vi "Lidar Camera System.vi"() -> ()   [LabVIEW 2017]
doc: "This example project provides a library of VIs that work together to wrap various ethernet packet sniffing functions available from WinPcap, a Windows packet capture program.\n\nNote: You must install WinPcap before running this example. You can download WinPcap from www.winpcap.org.\n\nThis VI reads ethernet packets. It outputs the raw data for the packet as a hexadecimal string. It also parses out the ethernet and IP header information, as well as timestamp information for each packet.\n\nThis VI also enumerates all the ethernet adapters on your system and allows you interactively to select between the various adapters.\n\nPlease note that this project is for demonstration purposes only. It was designed to demonstrate one method in which LabVIEW can be used to interface with external software utilities (such as WinPcap). NI Engineers can only address questions on how to call external code from LabVIEW, not the contents of each call demonstrated in this example. In addition, we cannot guarantee that the software will work with newer versions of the external software package."
uses:
  lvwpcap.lvlib
panel:
  in  "stop":bool
  in  "?":T1(tab)
  out "packets":i32
  out "raw data":string
  out "timestamp":cluster{"tv_sec":u32, "tv_usec":u32}
  in  "Adapters":i32(listbox)
  out "Packet Length":i32
  out "Stored Packet":string
  out "Discarded Packet":string
  out "Status":string
  out "Identifier":string
  out "Data Points":dbl[][](array[numeric])
  out "Z Vector":dbl[](array[numeric])
  out "Y Vector":dbl[](array[numeric])
  out "X Vector":dbl[](array[numeric])
  out "Reflectivity Vector":dbl[](array[numeric])
  out "X":dbl[](array[numeric])
  out "Y":dbl[](array[numeric])
  out "Z":dbl[](array[numeric])
  out "3D LIDAR Data":refnum<vi>(3d-picture)
  out "Colour Map":dbl[][](graph)
  out "Status 2":string
  out "Y Array":dbl[](array[numeric])
  out "Z Array":dbl[](array[numeric])
  out "X Array":dbl[](array[numeric])
  out "Size":i32
  # "See diagram for details."
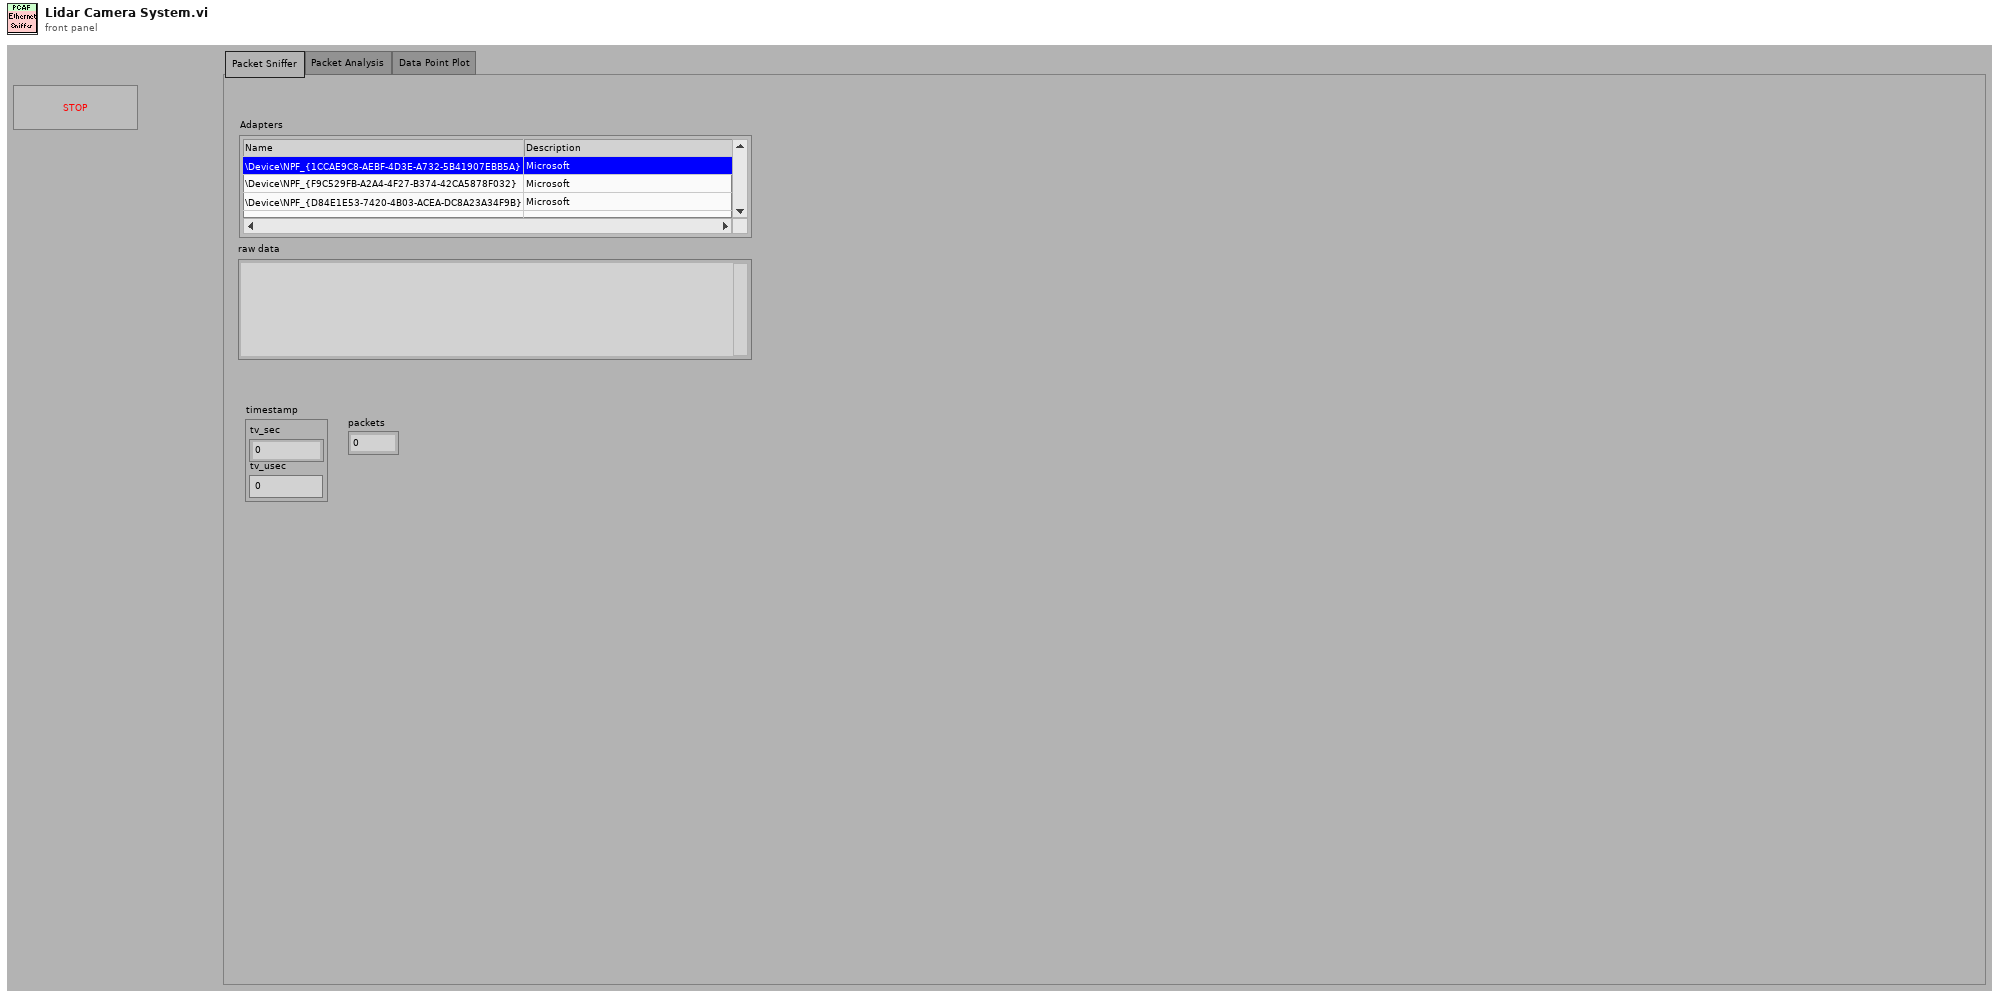
[diagram p1: front panel]
types:
  T1 = enum32{"Packet Sniffer", "Packet Analysis", "Data Point Plot"}
  T2 = enum16{"Store Values", "Check Array Size", "Plot Data", "Reinitialise Array"}
  T3 = enum16{"Check Data", "Check Identifier", "Convert to Hex", "Convert to XYZ", "Check Coords"}
  T4 = enum16{"Overall", "Per Primitive", "Per Vertex", "Binding Off"}
  T5 = typedef "LVRGBAColorTypeDef.ctl" = cluster{"Red":sgl, "Green":sgl, "Blue":sgl, "Alpha":sgl}
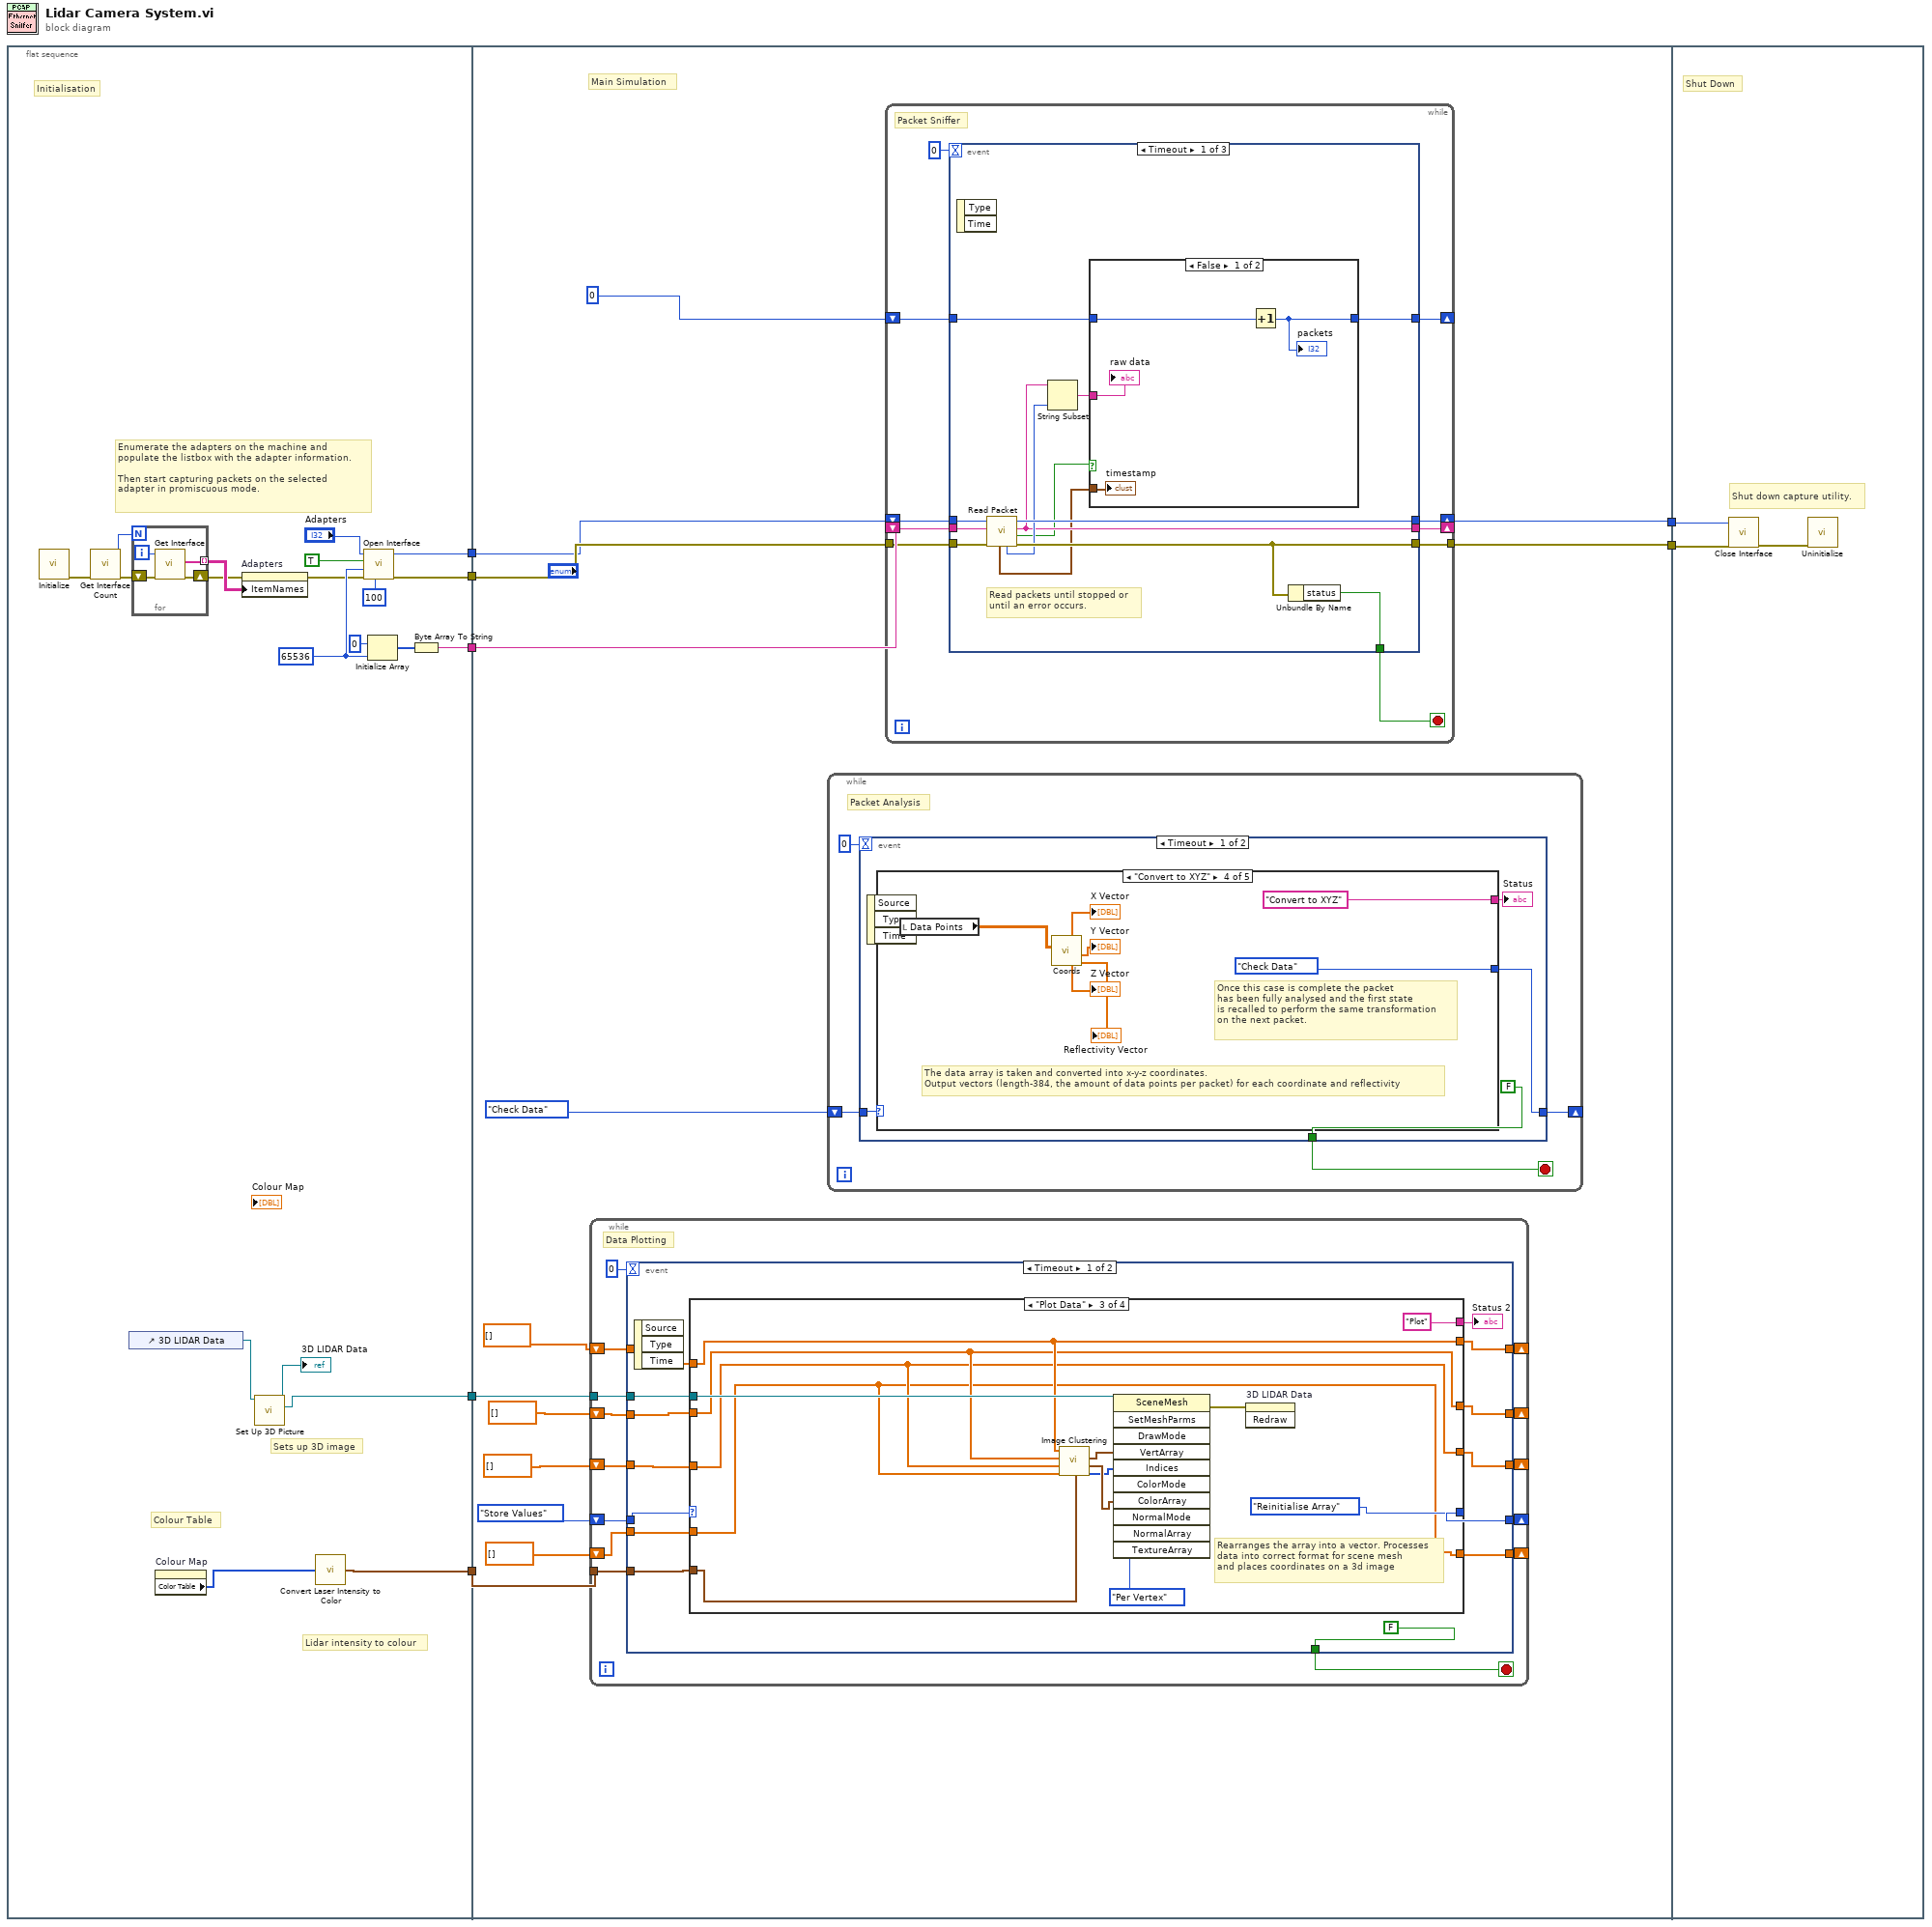
[diagram p0: block diagram]
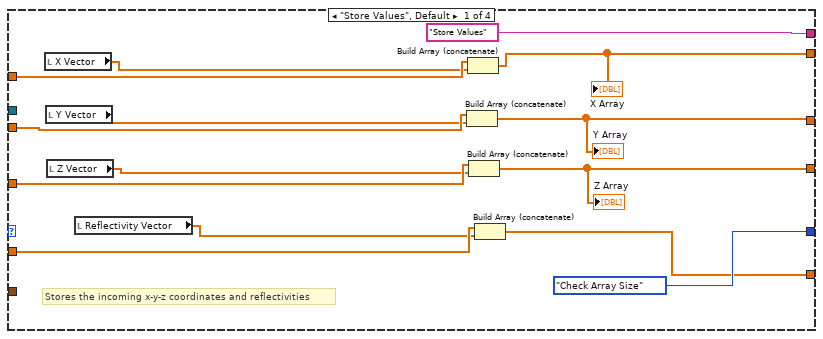
[diagram p2: hidden frame]
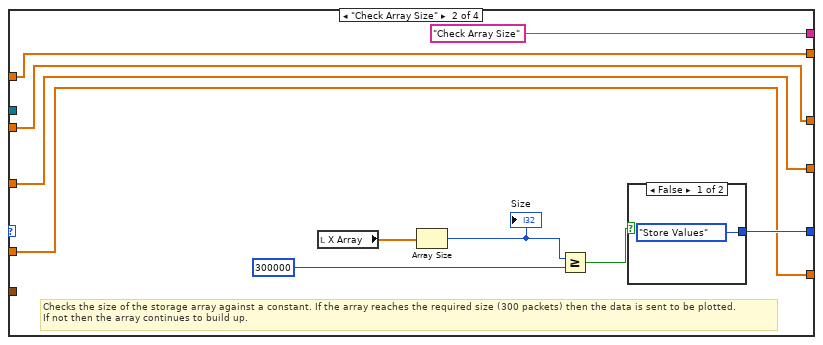
[diagram p3: hidden frame]
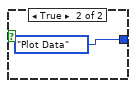
[diagram p4: hidden frame]
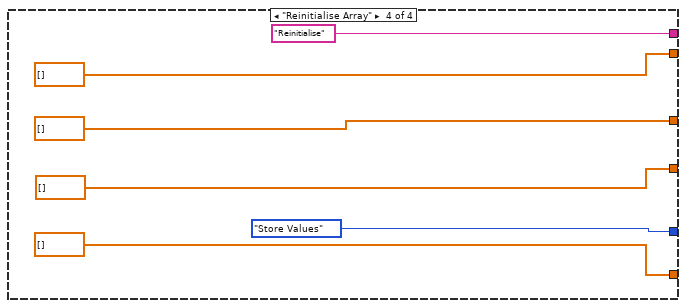
[diagram p5: hidden frame]
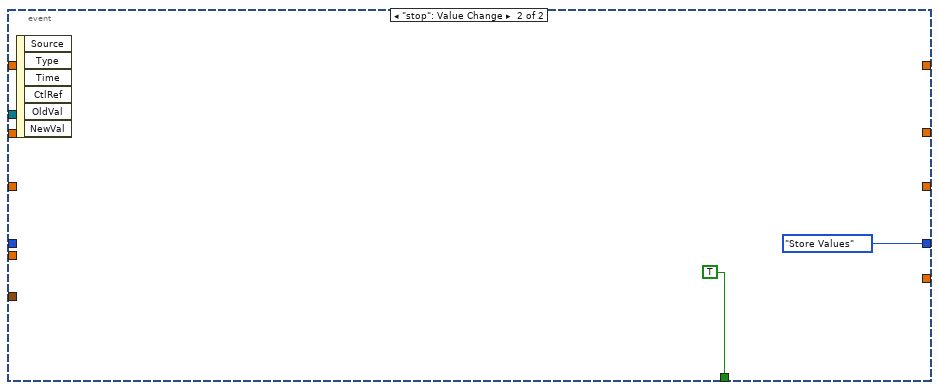
[diagram p6: hidden frame]
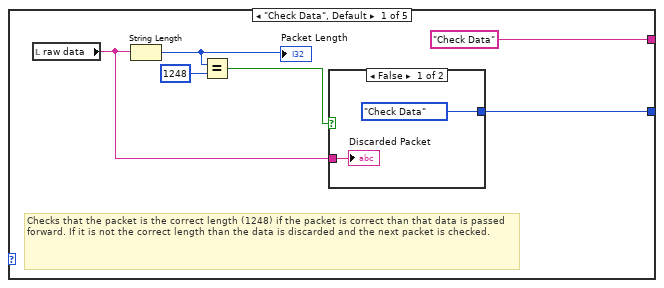
[diagram p7: hidden frame]
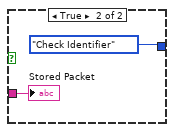
[diagram p8: hidden frame]
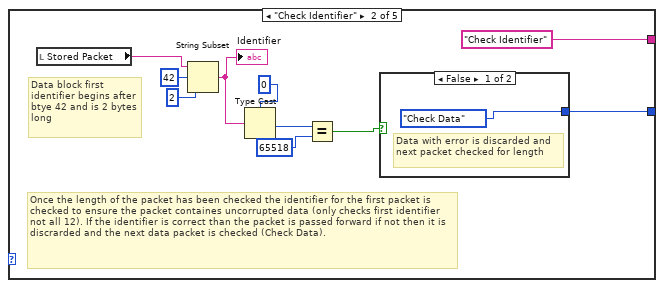
[diagram p9: hidden frame]
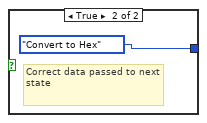
[diagram p10: hidden frame]
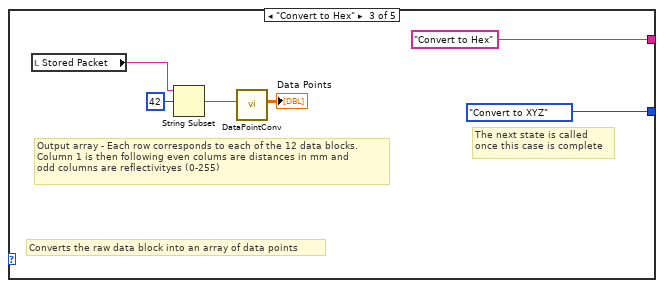
[diagram p11: hidden frame]
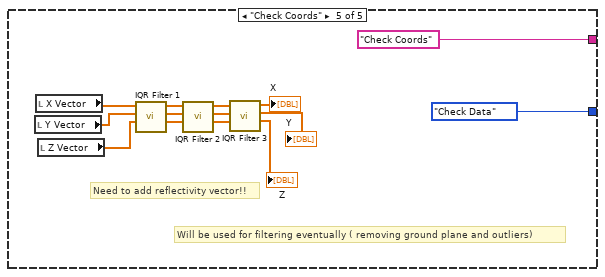
[diagram p12: hidden frame]
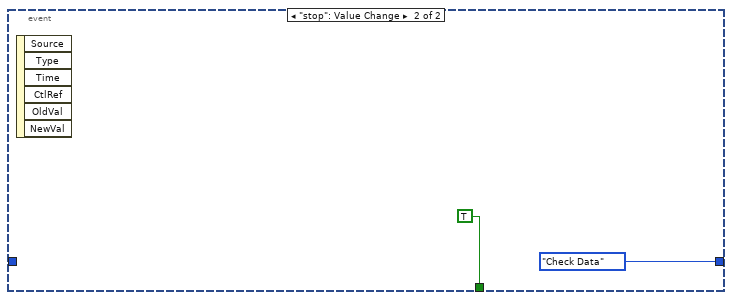
[diagram p13: hidden frame]
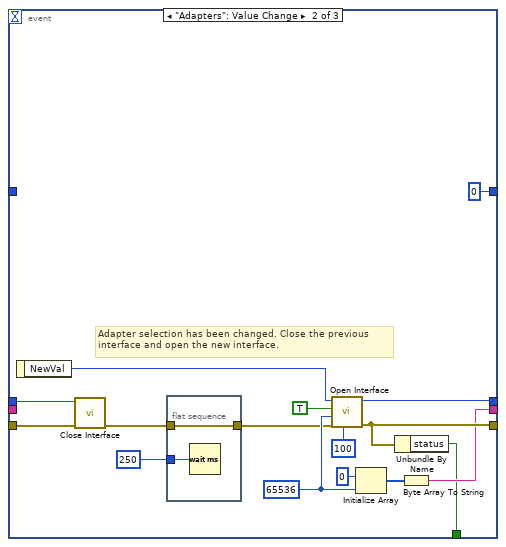
[diagram p15: hidden frame]
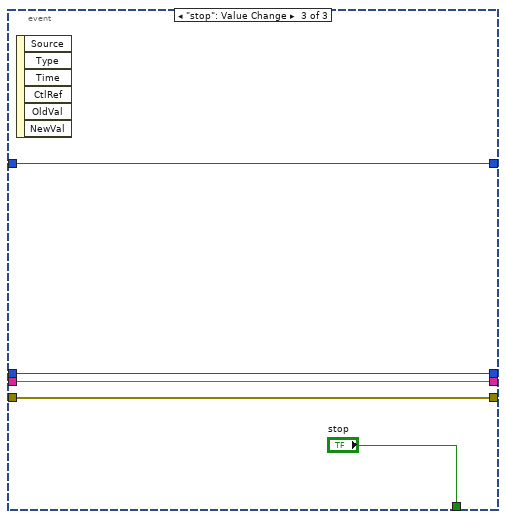
[diagram p16: hidden frame]
diagram:
  n1 = flat-sequence {
    tunnel: [w27] -> w7
    tunnel: [w26] -> w6
    tunnel: [w22] -> w5
    tunnel: [w12] -> w2
    tunnel: [w10] -> w1
    tunnel: w7 -> [w44]
    tunnel: w6 -> [w45]
    tunnel: w5 -> [w43]
    tunnel: [w42] -> w4
    tunnel: [w41] -> w3
    tunnel: w2 -> [w33]
    tunnel: w1 -> [w32]
    tunnel: w4 -> [w233]
    tunnel: w3 -> [w232]
    frame #0 {
      w25 = 65536 ("capture_size (65536)")
      # "Lidar intensity to colour"
      # "Sets up 3D image"
      # "Colour Table"
      # "Initialisation"
      # "Enumerate the adapters on the machine and\npopulate the listbox with the adapter information.\n\nThen start capturing packets on the selected\nadapter in promiscuous mode."
      n2 = call "Initialize.vi"() -> ("error out"=w20:errorcluster)  [unwired: 11 in]
      n3 = call "Get Interface Count.vi"("error in (no error)"=w20) -> ("error out"=w19:errorcluster, "count"=w18:i32)  [unwired: 9 in]
      n4 = control-ref of="3D LIDAR Data"() -> (w8:refnum<vi>)
      n5 = for {
        N: w18 -> [_]
        shift-right: [w30] -> w14
        shift-left: w19 -> [w31]
        tunnel: [w28] -> w16 mode=indexing
        i -> [w29]
        n6 = call "Get Interface.vi"("error in (no error)"=w31, "index"=w29) -> ("error out"=w30:errorcluster, "lvwpcap_interface_array"=w28:string[])  [unwired: 8 in]
      }
      n7 = property on="Colour Map" class="IntGraph (strict)"() -> ("Color Table"=w11:u32[])  [unwired: 2 in, 2 out]
      n8 = property on="Adapters" class="MCListbox (strict)"(error in=w14, "ItemNames"=w16) -> (error out=w13:errorcluster)  [unwired: 1 in, 1 out]
      n9 = call <instrlib>:"Set Up 3D Picture.vi"("3D Picture Control In"=w8) -> ("Mesh Out"=w10:refnum<vi>, "Scene Out"=→"3D LIDAR Data":refnum<vi>)  [unwired: 9 in]
      n10 = call <instrlib>:"Convert Laser Intensity to Color.vi"("Color Table"=w11) -> ("Color Array"=w12:T5[])  [unwired: 8 in]
      n11 = call "Open Interface.vi"("read_timeout (1000)"=100, "error in (no error)"=w13, "capture_size (65536)"=w25, "promiscuous mode (T)"=TRUE, "adapter (0)"="Adapters") -> ("error out"=w26:errorcluster, "pcap reference"=w27:u32)  [unwired: 5 in]
      n12 = Initialize Array(u8 0, w25) -> (w23:u8[])
      n13 = Byte Array To String(unsigned byte array=w23) -> (string=w22:string)
    }
    frame #1 {
      # "Main Simulation"
      n14 = while {
        shift-right: [w55] -> _
        shift-left: T2."Store Values" -> [w59]
        shift-right: [w49] -> _
        shift-left: dbl[] [] -> [w58]
        shift-right: [w48] -> _
        shift-left: dbl[] [] -> [w57]
        shift-right: [w47] -> _
        shift-left: dbl[] [] -> [w56]
        shift-right: [w46] -> _
        shift-left: dbl[] [] -> [w52]
        tunnel: w33 -> [w51]
        tunnel: w32 -> [w50]
        stop <- w54 stop-if-true
        # "Data Plotting"
        n15 = event shown="[0] Timeout" {
          selector: _ -> [_ _]
          dyn-events: _ -> [_ _]
          timeout: 0 -> [_ _]
          tunnel: w59 -> [w73 _]
          tunnel: w58 -> [w72 _]
          tunnel: w57 -> [w71 _]
          tunnel: w56 -> [w70 _]
          tunnel: [w69 T2."Store Values"] -> w55
          tunnel: [FALSE TRUE] -> w54
          tunnel: w52 -> [w66 _]
          tunnel: w51 -> [w65 _]
          tunnel: w50 -> [w64 _]
          tunnel: [w63 _] -> w49
          tunnel: [w62 _] -> w48
          tunnel: [w61 _] -> w47
          tunnel: [w60 _] -> w46
          event Timeout {
            n16 = event-data() -> ()  [unwired: 1 in, 3 out]
            n17 = case shown="\"Plot Data\"" w73 {
              tunnel: w72 -> [w85 w93 w103 _]
              tunnel: w71 -> [w83 w92 w102 _]
              tunnel: w70 -> [w82 w91 w101 _]
              tunnel: [w77 w93 w103 dbl[] []] -> w63
              tunnel: [w76 w92 w102 dbl[] []] -> w62
              tunnel: [w75 w91 w101 dbl[] []] -> w61
              tunnel: [T2."Check Array Size" w94 T2."Reinitialise Array" T2."Store Values"] -> w69
              tunnel: ["Store Values" "Check Array Size" "Plot" "Reinitialise"] -> w68
              tunnel: w66 -> [w80 w90 w100 _]
              tunnel: [w78 w90 w100 dbl[] []] -> w60
              tunnel: w65 -> [_ _ w110 _]
              tunnel: w64 -> [_ _ w109 _]
              frame "Store Values", Default {
                # "Stores the incoming x-y-z coordinates and reflectivities"
                n18 = local read "X Vector"() -> (w84:dbl[])
                n19 = local read "Y Vector"() -> (w74:dbl[])
                n20 = local read "Z Vector"() -> (w81:dbl[])
                n21 = local read "Reflectivity Vector"() -> (w79:dbl[])
                n22 = Build Array (concatenate)(w83, w74) -> (w76:dbl[])
                "Y Array" <- w76
                n23 = Build Array (concatenate)(w85, w84) -> (w77:dbl[])
                "X Array" <- w77
                n24 = Build Array (concatenate)(w82, w81) -> (w75:dbl[])
                "Z Array" <- w75
                n25 = Build Array (concatenate)(w80, w79) -> (w78:dbl[])
              }
              frame "Check Array Size" {
                # "Checks the size of the storage array against a constant. If the array reaches the required size (300 packets) then the data is sent to be plotted.\nIf not then the array continues to build up."
                n26 = local read "X Array"() -> (w89:dbl[])
                n27 = Array Size(array=w89) -> (size(s)=w88:i32)
                "Size" <- w88
                n28 = Greater Or Equal?(x=w88, y=300000) -> (x >= y?=w95:bool)
                n29 = case shown="False" w95 {
                  tunnel: [T2."Store Values" T2."Plot Data"] -> w94
                  frame False {
                  }
                  frame True {
                  }
                }
              }
              frame "Plot Data" {
                # "Rearranges the array into a vector. Processes\ndata into correct format for scene mesh\nand places coordinates on a 3d image"
                n30 = call "Image Clustering.vi"("Color Array"=w110, "Reflect"=w100, "Z"=w101, "Y"=w102, "X"=w103) -> ("Indicies"=w106:u32[], "Colour Coords"=w107:T5[], "XYZ Coords"=w108:cluster{"X":dbl, "Y":dbl, "Z":dbl}[])  [unwired: 4 in]
                n31 = invoke class="SceneMesh" method="SetMeshParms"(reference=w109, "VertArray"=w108, "Indices"=w106, "ColorMode"=T4."Per Vertex" ("Color Binding Mode"), "ColorArray"=w107) -> (error out=w104:errorcluster)  [unwired: 6 in, 10 out]
                n32 = invoke on="3D LIDAR Data" class="SceneGraphDisp (strict)" method="Redraw"(error in=w104) -> ()  [unwired: 2 in, 3 out]
              }
              frame "Reinitialise Array" {
              }
            }
            "Status 2" <- w68
          }
          event "stop": Value Change {
            n33 = event-data() -> ()  [unwired: 1 in, 6 out]
          }
        }
      }
      n34 = while {
        shift-right: [w123] -> _
        shift-left: T3."Check Data" -> [w124]
        stop <- w122 stop-if-true
        # "Packet Analysis"
        n35 = event shown="[0] Timeout" {
          selector: _ -> [_ _]
          dyn-events: _ -> [_ _]
          timeout: 0 -> [_ _]
          tunnel: w124 -> [w128 _]
          tunnel: [w127 T3."Check Data"] -> w123
          tunnel: [FALSE TRUE] -> w122
          event Timeout {
            n36 = event-data() -> ()  [unwired: 1 in, 3 out]
            n37 = case shown="\"Convert to XYZ\"" w128 {
              tunnel: [w130 w144 T3."Convert to XYZ" T3."Check Data" T3."Check Data"] -> w127
              tunnel: ["Check Data" "Check Identifier" "Convert to Hex" "Convert to XYZ" "Check Coords"] -> w126
              frame "Check Data", Default {
                # "Checks that the packet is the correct length (1248) if the packet is correct than that data is passed forward. If it is not the correct length than the data is discarded and the next packet is checked."
                n38 = local read "raw data"() -> (w131:string)
                n39 = String Length(string=w131) -> (length=w134:i32)
                "Packet Length" <- w134
                n40 = Equal?(x=w134, y=1248) -> (x = y?=w132:bool)
                n41 = case shown="False" w132 {
                  tunnel: w131 -> [w136 w138]
                  tunnel: [T3."Check Data" T3."Check Identifier"] -> w130
                  frame False {
                    "Discarded Packet" <- w136
                  }
                  frame True {
                    "Stored Packet" <- w138
                  }
                }
              }
              frame "Check Identifier" {
                # "Data block first identifier begins after btye 42 and is 2 bytes long"
                # "Once the length of the packet has been checked the identifier for the first packet is checked to ensure the packet containes uncorrupted data (only checks first identifier not all 12). If the identifier is correct than the packet is passed forward if not then it is discrarded and the next data packet is checked (Check Data)."
                n42 = local read "Stored Packet"() -> (w148:string)
                n43 = String Subset(string=w148, offset (0)=42, length (rest)=2 ("length (rest)")) -> (substring=w142:string)
                "Identifier" <- w142
                n44 = Type Cast(type=u16 0, x=w142) -> (*(type *) &x=w140:u16)
                n45 = Equal?(x=w140, y=u16 65518) -> (x = y?=w145:bool)
                n46 = case shown="False" w145 {
                  tunnel: [T3."Check Data" T3."Convert to Hex"] -> w144
                  frame False {
                    # "Data with error is discarded and next packet checked for length"
                  }
                  frame True {
                    # "Correct data passed to next state"
                  }
                }
              }
              frame "Convert to Hex" {
                # "The next state is called \nonce this case is complete"
                # "Output array - Each row corresponds to each of the 12 data blocks.\nColumn 1 is then following even colums are distances in mm and \nodd columns are reflectivityes (0-255)"
                # "Converts the raw data block into an array of data points"
                n47 = local read "Stored Packet"() -> (w154:string)
                n48 = String Subset(string=w154, offset (0)=42) -> (substring=w152:string)  [unwired: 1 in]
                n49 = call "DataPointConv.vi"("Stored Data"=w152) -> ("Data Points"=→"Data Points":dbl[][])  [unwired: 10 in]
              }
              frame "Convert to XYZ" {
                # "Once this case is complete the packet\nhas been fully analysed and the first state\nis recalled to perform the same transformation \non the next packet."
                # "The data array is taken and converted into x-y-z coordinates.\nOutput vectors (length-384, the amount of data points per packet) for each coordinate and reflectivity"
                n50 = local read "Data Points"() -> (w161:dbl[][])
                n51 = call "Coords.vi"("Data Points"=w161) -> ("Reflectivity Vector"=→"Reflectivity Vector":dbl[], "Y Vector"=→"Y Vector":dbl[], "Z Vector"=→"Z Vector":dbl[], "X Vector"=→"X Vector":dbl[])  [unwired: 7 in]
              }
              frame "Check Coords" {
                # "Need to add reflectivity vector!!"
                # "Will be used for filtering eventually ( removing ground plane and outliers)"
                n52 = local read "Y Vector"() -> (w174:dbl[])
                n53 = local read "X Vector"() -> (w175:dbl[])
                n54 = local read "Z Vector"() -> (w173:dbl[])
                n55 = call "IQR Filter 1.vi"("Z Values"=w173, "Y Values"=w174, "X Values"=w175) -> ("Z Vector"=w170:dbl[], "Y Vector"=w171:dbl[], "X Value"=w172:dbl[])  [unwired: 6 in]
                n56 = call "IQR Filter 2.vi"("Z Values"=w170, "Y Values"=w171, "X Values"=w172) -> ("Z Vector"=w167:dbl[], "Y Vector"=w168:dbl[], "X Value"=w169:dbl[])  [unwired: 6 in]
                n57 = call "IQR Filter 3.vi"("Z Values"=w167, "Y Values"=w168, "X Values"=w169) -> ("Z Vector"=→"Z":dbl[], "Y Vector"=→"Y":dbl[], "X Value"=→"X":dbl[])  [unwired: 6 in]
              }
            }
            "Status" <- w126
          }
          event "stop": Value Change {
            n58 = event-data() -> ()  [unwired: 1 in, 6 out]
          }
        }
      }
      n59 = while {
        tunnel: w45 -> [w188]
        tunnel: [w187] -> w42
        shift-right: [w186] -> w41
        shift-left: w44 -> [w189]
        shift-right: [w184] -> _
        shift-left: w43 -> [w185]
        shift-right: [w182] -> _
        shift-left: 0 -> [w183]
        stop <- w180 stop-if-true
        # "Packet Sniffer"
        n60 = event shown="[0] Timeout" {
          selector: _ -> [_ _ _]
          dyn-events: _ -> [_ _ _]
          timeout: 0 -> [_ _ _]
          tunnel: w189 -> [w202 w210 w229]
          tunnel: w188 -> [w201 w222 w227]
          tunnel: [w200 w223 w227] -> w187
          tunnel: [w199 w220 w229] -> w186
          tunnel: w185 -> [w198 _ w228]
          tunnel: [w196 w215 w228] -> w184
          tunnel: w183 -> [w193 _ w226]
          tunnel: [w192 0 w226] -> w182
          tunnel: [w191 w213 "stop"] -> w180
          event Timeout {
            # "Read packets until stopped or\nuntil an error occurs."
            n61 = event-data() -> ()  [unwired: 1 in, 2 out]
            n62 = call "Read Packet.vi"("error in (no error)"=w201, "capture_data"=w198, "pcap reference"=w202) -> ("error out"=w200:errorcluster, "timed out"=w194:bool, "capture_data out"=w196:string, "pcap reference out"=w199:u32, "capture_len"=w197:u32, "timestamp"=w190:cluster{"tv_sec":u32, "tv_usec":u32})  [unwired: 3 in]
            n63 = String Subset(string=w196, length (rest)=w197) -> (substring=w195:string)  [unwired: 1 in]
            n64 = case shown="False" w194 {
              tunnel: w195 -> [w206 _]
              tunnel: w190 -> [w205 _]
              tunnel: w193 -> [w204 w207]
              tunnel: [w203 w207] -> w192
              frame False {
                n65 = Increment(x=w204) -> (x+1=w203:i32)
                "packets" <- w203
                "raw data" <- w206
                "timestamp" <- w205
              }
              frame True {
                # "timed out"
              }
            }
            n66 = Unbundle By Name(w200) -> ("status"=w191:bool)
          }
          event "Adapters": Value Change {
            w216 = 65536 ("capture_size (65536)")
            # "Adapter selection has been changed. Close the previous\ninterface and open the new interface."
            n67 = event-data() -> ("NewVal"=w221:i32)  [unwired: 1 in]
            n68 = call "Close Interface.vi"("error in (no error)"=w222, "pcap reference"=w210) -> ("error out"=w209:errorcluster)  [unwired: 9 in]
            n69 = flat-sequence {
              tunnel: w209 -> [w225]
              tunnel: [w225] -> w208
              tunnel: u32 250 ("milliseconds to wait") -> [w224]
              frame #0 {
                n70 = Wait (ms)(milliseconds to wait=w224) -> ()  [unwired: 1 out]
              }
            }
            n71 = call "Open Interface.vi"("read_timeout (1000)"=100, "error in (no error)"=w208, "capture_size (65536)"=w216, "promiscuous mode (T)"=TRUE, "adapter (0)"=w221) -> ("error out"=w223:errorcluster, "pcap reference"=w220:u32)  [unwired: 5 in]
            n72 = Initialize Array(u8 0, w216) -> (w218:u8[])
            n73 = Unbundle By Name(w223) -> ("status"=w213:bool)
            n74 = Byte Array To String(unsigned byte array=w218) -> (string=w215:string)
          }
          event "stop": Value Change {
            n75 = event-data() -> ()  [unwired: 1 in, 6 out]
          }
        }
      }
    }
    frame #2 {
      # "Shut Down"
      # "Shut down capture utility."
      n76 = call "Close Interface.vi"("error in (no error)"=w233, "pcap reference"=w232) -> ("error out"=w231:errorcluster)  [unwired: 9 in]
      n77 = call "Uninitialize.vi"("error in (no error)"=w231) -> ()  [unwired: 10 in, 1 out]
    }
  }
